vi "Get Frame Signals.vi"(5 "Limit?":bool, 7 "Address":u8, 8 "error in":errorcluster, 9 "Parent Tag":string, 10 "Tree Reference":refnum<vi>, 11 "Frms":refnum<k21>[](array[refnum])) -> (0 "error out":errorcluster, 2 "Tree Reference Out":refnum<vi>)   [LabVIEW 2013, in "J1939 Addon System Explorer.lvlib"]
uses:
  J1939 Addon System Explorer.lvlib
  <resource>/objmgr/xnet.rc
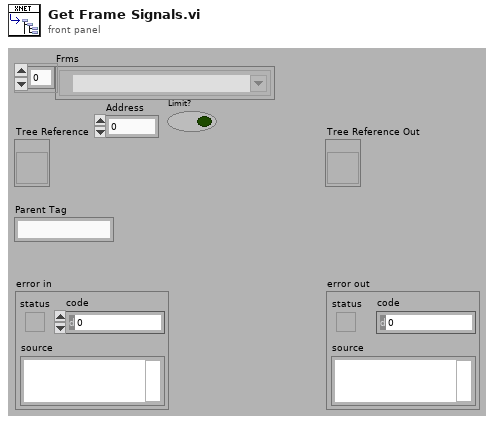
[diagram p1: front panel]
types:
  T1 = enum16{"open", "replace", "create", "open or create", "replace or create", "replace or create with confirmation"}
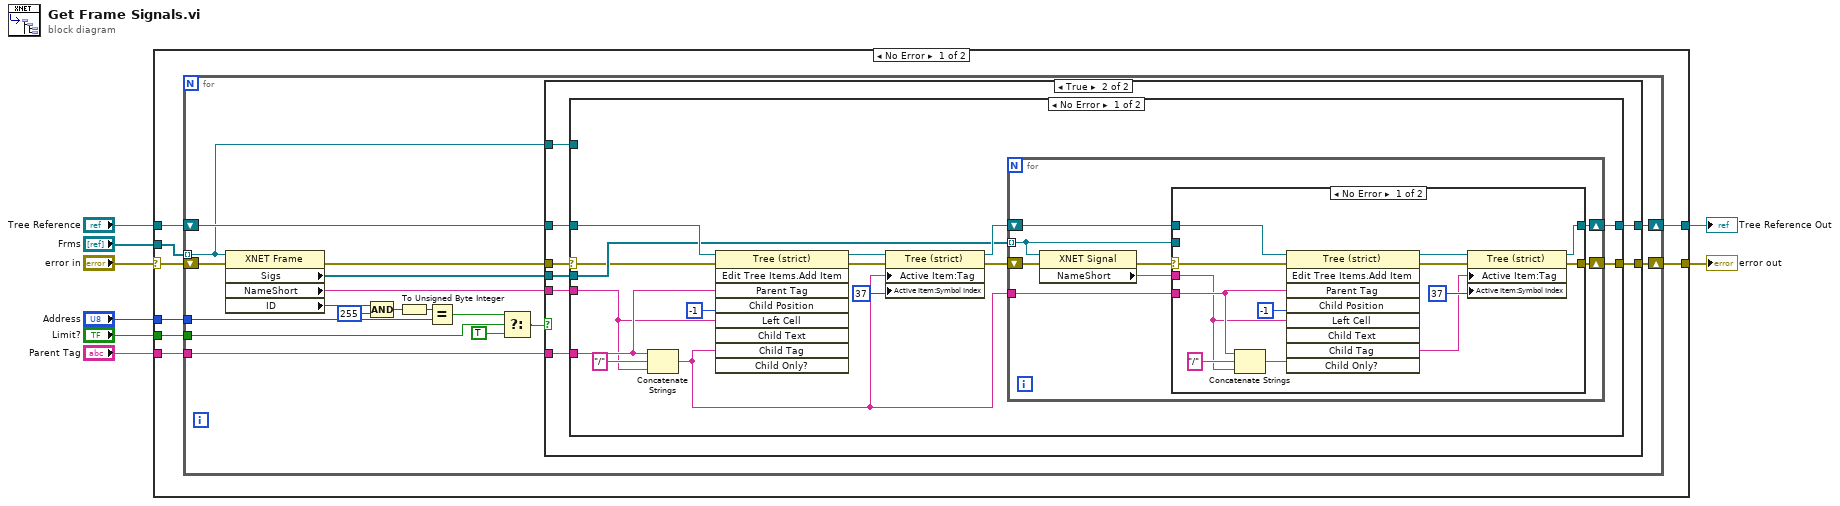
[diagram p0: block diagram]
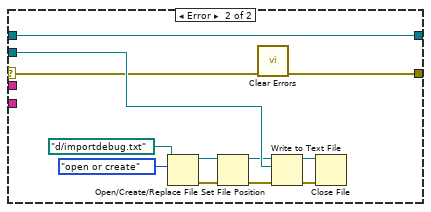
[diagram p3: hidden frame]
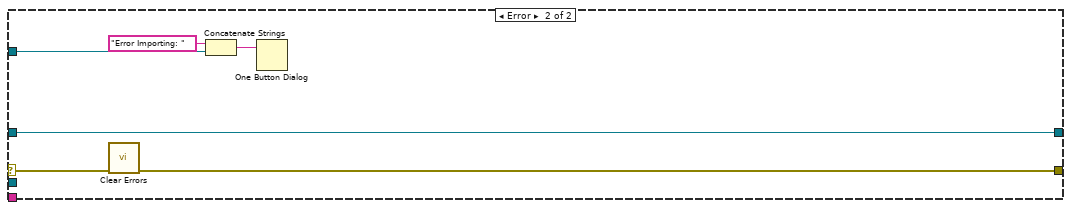
[diagram p4: hidden frame]
diagram:
  n1 = case shown="No Error" "error in" {
    selector: "error in" -> [w13 w99]
    tunnel: [w16 w99] -> w8
    tunnel: "Frms" -> [w11 _]
    tunnel: "Tree Reference" -> [w15 w98]
    tunnel: "Parent Tag" -> [w14 _]
    tunnel: [w12 w98] -> w3
    tunnel: "Address" -> [w10 _]
    tunnel: "Limit?" -> [w9 _]
    frame No Error {
      n2 = for {
        tunnel: w11 -> [w26] mode=indexing
        shift-right: [w29] -> w16
        shift-left: w13 -> [w34]
        tunnel: w14 -> [w32]
        shift-right: [w31] -> w12
        shift-left: w15 -> [w33]
        tunnel: w10 -> [w19]
        tunnel: w9 -> [w18]
        n3 = property class="XNET Frame"(reference=w26, error in=w34) -> (error out=w27:errorcluster, "Sigs"=w30:refnum<k21>[], "NameShort"=w28:string, "ID"=w21:u32)  [unwired: 1 out]
        n4 = Compound Arithmetic op=AND(w21, u32 255 ("value")) -> (w20:u32)
        n5 = To Unsigned Byte Integer(number=w20) -> (unsigned 8bit integer=w17:u8)
        n6 = Equal?(x=w17, y=w19) -> (x = y?=w25:bool)
        n7 = Select(t=w25, s=w18, f=TRUE) -> (s? t:f=w23:bool)
        n8 = case shown="True" w23 {
          tunnel: w33 -> [w36 w44]
          tunnel: w32 -> [_ w43]
          tunnel: [w36 w42] -> w31
          tunnel: w30 -> [_ w41]
          tunnel: [w35 w40] -> w29
          tunnel: w28 -> [_ w39]
          tunnel: w27 -> [w35 w38]
          tunnel: w26 -> [_ w37]
          frame False {
          }
          frame True {
            n9 = case shown="No Error" w38 {
              selector: w38 -> [w45 w94]
              tunnel: w44 -> [w59 w92]
              tunnel: w43 -> [w56 _]
              tunnel: [w55 w92] -> w42
              tunnel: w41 -> [w48 _]
              tunnel: [w47 w93] -> w40
              tunnel: w39 -> [w46 _]
              tunnel: w37 -> [_ w97]
              frame No Error {
                n10 = Concatenate Strings(w56, "/" ("string"), w46) -> (w49:string)
                n11 = invoke on="Invoke Node" class="Tree (strict)" method="Edit Tree Items.Add Item"(reference=w59, error in=w45, "Parent Tag"=w56, "Child Position"=-1, "Left Cell"=w46, "Child Tag"=w49) -> (reference out=w52:refnum<vi>, error out=w53:errorcluster)  [unwired: 3 in, 7 out]
                n12 = property class="Tree (strict)"(reference=w52, error in=w53, "Active Item:Tag"=w49, "Active Item:Symbol Index"=37) -> (reference out=w50:refnum<vi>, error out=w51:errorcluster)
                n13 = for {
                  tunnel: w48 -> [w60] mode=indexing
                  shift-right: [w62] -> w47
                  shift-left: w51 -> [w67]
                  tunnel: w49 -> [w65]
                  shift-right: [w63] -> w55
                  shift-left: w50 -> [w66]
                  n14 = property class="XNET Signal"(reference=w60, error in=w67) -> (error out=w61:errorcluster, "NameShort"=w64:string)  [unwired: 1 out]
                  n15 = case shown="No Error" w61 {
                    selector: w61 -> [w68 w89]
                    tunnel: w66 -> [w79 w91]
                    tunnel: w65 -> [w77 _]
                    tunnel: w64 -> [w76 _]
                    tunnel: [w71 w91] -> w63
                    tunnel: [w69 w88] -> w62
                    tunnel: w60 -> [_ w90]
                    frame No Error {
                      n16 = Concatenate Strings(w77, "/" ("string"), w76) -> (w70:string)
                      n17 = invoke on="Invoke Node" class="Tree (strict)" method="Edit Tree Items.Add Item"(reference=w79, error in=w68, "Parent Tag"=w77, "Child Position"=-1, "Left Cell"=w76, "Child Tag"=w70) -> (reference out=w72:refnum<vi>, error out=w73:errorcluster)  [unwired: 3 in, 7 out]
                      n18 = property class="Tree (strict)"(reference=w72, error in=w73, "Active Item:Tag"=w70, "Active Item:Symbol Index"=37) -> (reference out=w71:refnum<vi>, error out=w69:errorcluster)
                    }
                    frame Error {
                      n19 = Open/Create/Replace File(file path (use dialog)=path "d:/importdebug.txt", operation (0:open)=T1."open or create") -> (refnum out=w85:refnum<file>, error out=w86:errorcluster)  [unwired: 4 in, 1 out]
                      n20 = Set File Position(refnum=w85, error in=w86) -> (refnum out=w84:refnum<file>, error out=w83:errorcluster)  [unwired: 2 in]
                      n21 = call <vilib>:"Clear Errors.vi"("error in (no error)"=w89) -> ("error out"=w88:errorcluster)  [unwired: 6 in]
                      n22 = Write to Text File(file (use dialog)=w84, text=w90, error in=w83) -> (refnum out=w81:refnum<file>, error out=w82:errorcluster)  [unwired: 1 in, 1 out]
                      n23 = Close File(refnum=w81, error in=w82) -> ()  [unwired: 2 out]
                    }
                  }
                }
              }
              frame Error {
                n24 = call <vilib>:"Clear Errors.vi"("error in (no error)"=w94) -> ("error out"=w93:errorcluster)  [unwired: 6 in]
                n25 = Concatenate Strings("Error Importing: " ("string"), w97) -> (w95:string)
                n26 = One Button Dialog(message=w95) -> ()  [unwired: 1 in, 1 out]
              }
            }
          }
        }
      }
    }
    frame Error {
    }
  }
  "error out" <- w8
  "Tree Reference Out" <- w3
